vi "LSCI 370 Config Control Mode.vi"(0 "VISA session":refnum<visa-resource-name>, 1 "Setpoint Units (0: Kelvin)":u16(ring) items=["Kelvin", "Ohms"], 2 "Setpoint Change\nPause Time (25)":i32=25 min=1 max=255 step=1, 5 "Control Mode (0: Closed Loop PID)":u16(ring) items=["Closed Loop PID", "Zone Tuning", "Open Loop", "Off"], 7 "Channel (1)":i32=1 min=1 max=16 step=1, 9 "Filtered Readings (0: Unfiltered)":u16(ring) items=["Unfiltered", "Filtered"], 11 "error in (no error)":errorcluster, 12 "Heater Output Display (0: Current)":u16(ring) items=["Current", "Power"], 13 "Heater Resistance (100.00)":dbl=100.0 min=1.0 max=100000.0 step=0.01 format="%.2f", 14 "Maximum Heater Range (0: 31.6 uA)":u16(ring) items=["31.6 uA", "100 uA", "316 uA", "1.00 mA", "3.16 mA", "10.0 mA", "31.6 mA", "100 mA"]) -> (4 "dup VISA session":refnum<visa-resource-name>, 15 "error out":errorcluster)   [LabVIEW 2018]
doc: "This VI selects the temperature control mode and configures the parameters of temperature control."
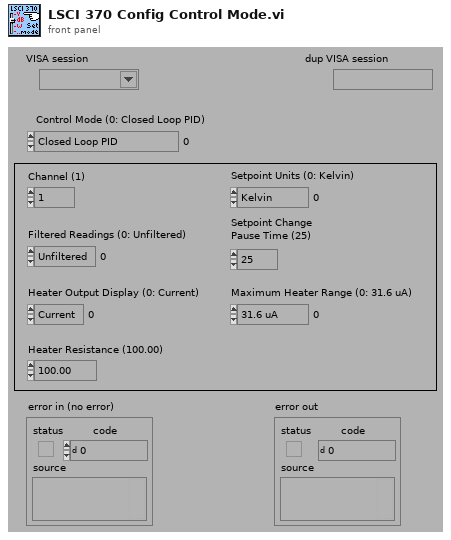
[diagram p1: front panel]
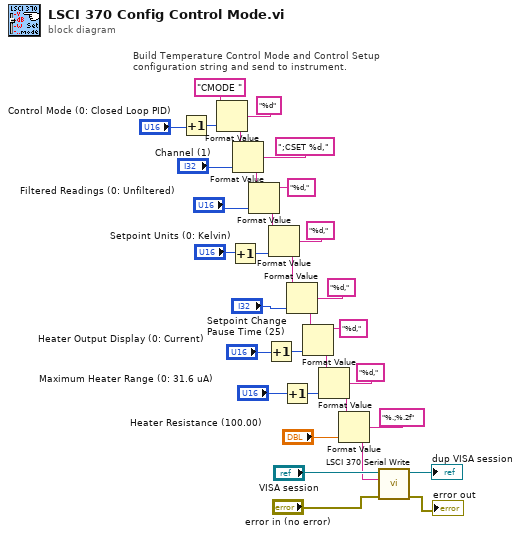
[diagram p0: block diagram]
diagram:
  # "Build Temperature Control Mode and Control Setup\nconfiguration string and send to instrument."
  n1 = Increment(x="Control Mode (0: Closed Loop PID)") -> (x+1=w27:u16)
  n2 = Format Value(string ("")="CMODE ", format string="%d", value (0)=w27) -> (output string=w17:string)
  n3 = Increment(x="Setpoint Units (0: Kelvin)") -> (x+1=w31:u16)
  n4 = Format Value(string ("")=w17, format string=";CSET %d,", value (0)="Channel (1)") -> (output string=w14:string)
  n5 = Format Value(string ("")=w14, format string="%d,", value (0)="Filtered Readings (0: Unfiltered)") -> (output string=w12:string)
  n6 = Increment(x="Heater Output Display (0: Current)") -> (x+1=w8:u16)
  n7 = Format Value(string ("")=w12, format string="%d,", value (0)=w31) -> (output string=w28:string)
  n8 = Increment(x="Maximum Heater Range (0: 31.6 uA)") -> (x+1=w4:u16)
  n9 = Format Value(string ("")=w28, format string="%d,", value (0)="Setpoint Change\nPause Time (25)") -> (output string=w10:string)
  n10 = Format Value(string ("")=w10, format string="%d,", value (0)=w8) -> (output string=w6:string)
  n11 = Format Value(string ("")=w6, format string="%d,", value (0)=w4) -> (output string=w2:string)
  n12 = Format Value(string ("")=w2, format string="%.;%.2f", value (0)="Heater Resistance (100.00)") -> (output string=w21:string)
  n13 = call "LSCI 370 Serial Write.vi"("error in (no error)"="error in (no error)", "Write Buffer (\"\")"=w21, "VISA session"="VISA session") -> ("error out"=→"error out":errorcluster, "dup VISA session"=→"dup VISA session":refnum<visa-resource-name>)  [unwired: 6 in, 1 out]
